vi "Config_OpenMake.vi"(8 "error in (no error)":errorcluster, 11 "Config Path":path) -> (0 "error out":errorcluster, 3 "File Path":path)   [LabVIEW 2021]
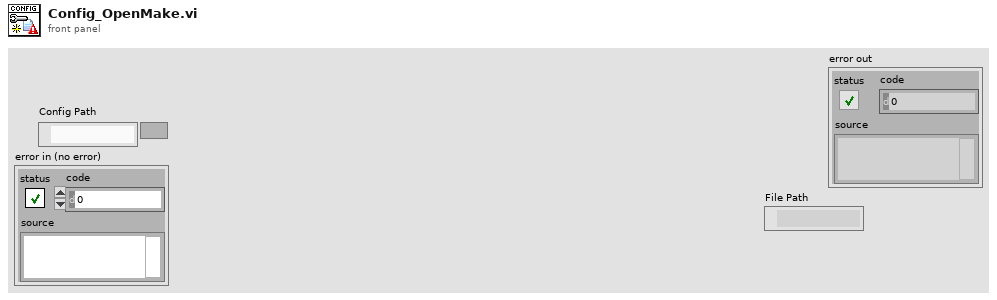
[diagram p1: front panel]
types:
  T1 = enum16{"open", "replace", "create", "open or create", "replace or create", "replace or create with confirmation"}
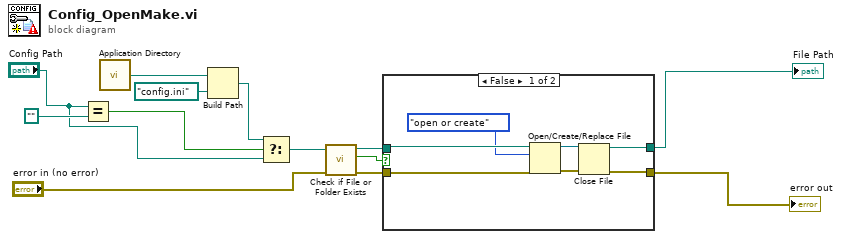
[diagram p0: block diagram]
diagram:
  n1 = Equal?(x="Config Path", y=path "") -> (x = y?=w12:bool)
  n2 = call <vilib>:"Application Directory.vi"() -> ("Application Directory"=w10:path)
  n3 = Build Path(base path=w10, name or relative path=path "config.ini") -> (appended path=w8:path)
  n4 = Select(t=w8, s=w12, f="Config Path") -> (s? t:f=w7:path)
  n5 = call <vilib>:"Check if File or Folder Exists.vi"("error in (no error)"="error in (no error)", "path"=w7) -> ("error out"=w3:errorcluster, "file or folder exists?"=w4:bool, "dup path"=w5:path)  [unwired: 7 in]
  n6 = case shown="False" w4 {
    tunnel: w5 -> [w20 w21]
    tunnel: w3 -> [w18 w22]
    tunnel: [w15 w22] -> w2
    tunnel: [w14 w21] -> w1
    frame False {
      n7 = Open/Create/Replace File(file path (use dialog)=w20, error in=w18, operation (0:open)=T1."open or create") -> (refnum out=w17:refnum<file>, error out=w16:errorcluster)  [unwired: 3 in, 1 out]
      n8 = Close File(refnum=w17, error in=w16) -> (path=w14:path, error out=w15:errorcluster)
    }
    frame True {
    }
  }
  "error out" <- w2
  "File Path" <- w1
